vi "Arrange VIWin - Get FP Controls Max Bottom.vi"(0 "controls":refnum<vi>[](array[refnum]), 11 "error in":errorcluster) -> (4 "max bottom":i16, 15 "error out":errorcluster)   [LabVIEW 2015, in "Arrange VI Window.lvlib"]
uses:
  Arrange VI Window.lvlib
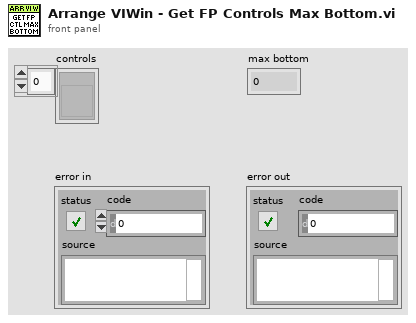
[diagram p1: front panel]
types:
  T1 = typedef "LVRectTypeDef.ctl" = cluster{"Left":i16, "Top":i16, "Right":i16, "Bottom":i16}
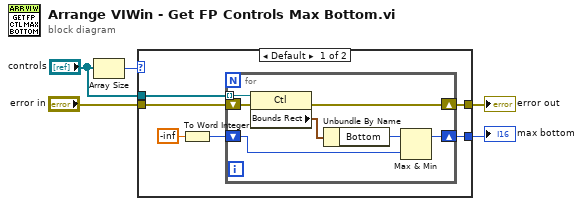
[diagram p0: block diagram]
diagram:
  n1 = Array Size(array="controls") -> (size(s)=w3:i32)
  n2 = case shown="Default" w3 {
    tunnel: "error in" -> [w9 w19]
    tunnel: [w8 w19] -> w2
    tunnel: "controls" -> [w7 _]
    tunnel: [w6 _] -> w4
    frame Default {
      n3 = To Word Integer(number=-inf) -> (16bit integer=w10:i16)
      n4 = for {
        shift-right: [w17] -> w8
        shift-left: w9 -> [w18]
        shift-right: [w14] -> w6
        shift-left: w10 -> [w13]
        tunnel: w7 -> [w12] mode=indexing
        n5 = property class="Ctl"(reference=w12, error in=w18) -> (error out=w17:errorcluster, "Bounds Rect"=w16:T1)  [unwired: 1 out]
        n6 = Unbundle By Name(w16) -> ("Bottom"=w15:i16)
        n7 = Max & Min(x=w15, y=w13) -> (max(x,y)=w14:i16)  [unwired: 1 out]
      }
    }
    frame 0 {
    }
  }
  "max bottom" <- w4
  "error out" <- w2
